vi "Time Estimate.vi"(8 "error in (no error)":errorcluster, 9 "expmode":i32, 10 "scantype":T1(ring), 11 "Pulse Gen Scan.lvclass":refnum<class "Pulse Gen Scan.lvclass">) -> (0 "error out":errorcluster, 1 "Time Estimate":string, 2 "time":dbl[unit], 3 "Pulse Gen Scan.lvclass":refnum<class "Pulse Gen Scan.lvclass">)   [LabVIEW 2009, in "Pulse Gen Scan.lvclass"]
uses:
  Pulse Gen Scan.lvclass
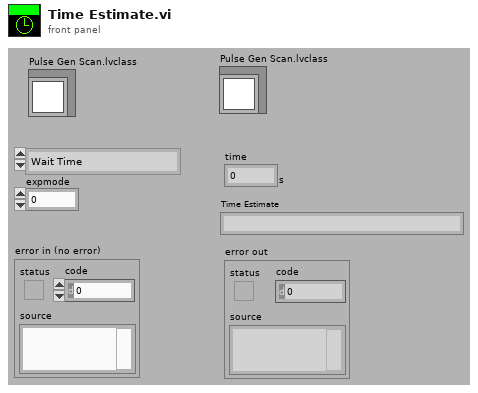
[diagram p1: front panel]
types:
  T1 = enum16{"Wait Time", "Pulse Width", "Wavelength", "Magnetic Field", "rf Scan"}
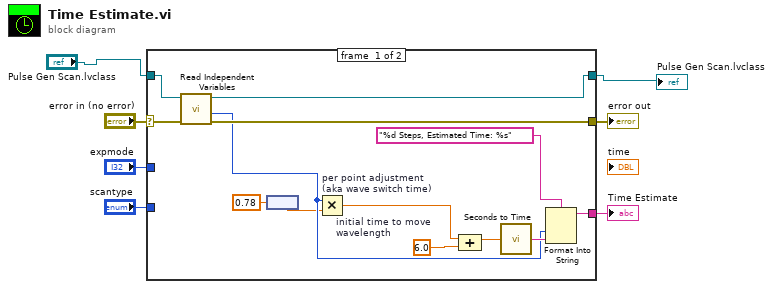
[diagram p0: block diagram]
diagram:
  n1 = case shown="No Error" "error in (no error)" {
    selector: "error in (no error)" -> [w17 w21]
    tunnel: [w13 _] -> w3
    tunnel: "expmode" -> [_ _]
    tunnel: "scantype" -> [_ _]
    tunnel: [w18 w22] -> w1
    tunnel: "Pulse Gen Scan.lvclass" -> [w19 w22]
    tunnel: [w20 w21] -> w5
    frame #0 {
      w11 = dbl[unit] 6.0  # initial time to move wavelength
      n2 = call-dynamic "Read Independent Variables.vi"("error in (no error)"=w17, "Scanner.lvclass in"=w19) -> ("error out"=w20:errorcluster, "size"=w14:i32, "Scanner.lvclass out"=w18:refnum<class "Pulse Gen Scan.lvclass">)  [unwired: 7 out]
      n3 = node(0.78) -> (w9:dbl[unit])
      n4 = Multiply "per point adjustment\n(aka wave switch time)"(x=w14, y=w9) -> (x*y=w12:dbl[unit])
      n5 = Compound Arithmetic op=ADD(w12, w11) -> (w8:dbl[unit])
      n6 = call "Seconds to Time.vi"("Seconds"=w8) -> ("Time"=w15:string)
      n7 = Format Into String(format string="%d Steps, Estimated Time: %s", w14, w15) -> (resulting string=w13:string)  [unwired: 2 in, 1 out]
    }
    frame #1 {
    }
  }
  "error out" <- w5
  "Time Estimate" <- w3
  "Pulse Gen Scan.lvclass" <- w1
